vi "push_number.vi"(8 "error in (no error)":errorcluster, 10 "value":dbl, 11 "Lua in":refnum<class "Lua.lvclass">) -> (0 "error out":errorcluster, 3 "Lua out":refnum<class "Lua.lvclass">)   [LabVIEW 2020, in "Lua for LabVIEW.lvlib" / "Lua.lvclass"]
doc: "Push a numeric value to the Lua stack."
uses:
  Lua.lvclass
  Lua.lvclass/Lua.ctl
  lib/lua.dll/types/lua_error_code_offset.vi
  <vilib>/Utility/error.llb/Error Cluster From Error Code.vi
  lib/lua.dll/lua_pushnumber.vi
  lib/lua.dll/lua.dll.lvlib
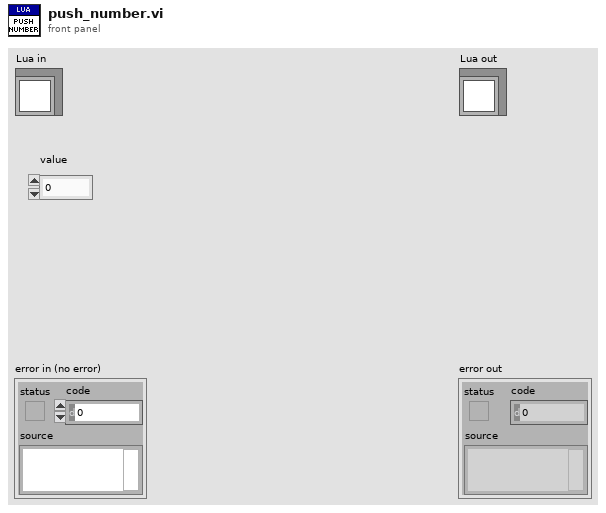
[diagram p1: front panel]
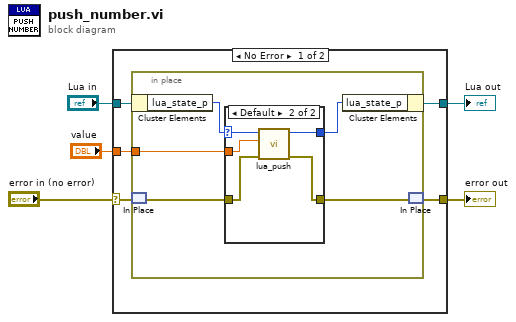
[diagram p0: block diagram]
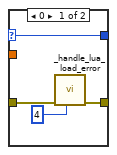
[diagram p2: hidden frame]
diagram:
  n1 = case shown="No Error" "error in (no error)" {
    selector: "error in (no error)" -> [w7 w26]
    tunnel: [w8 w26] -> w4
    tunnel: [w9 w25] -> w2
    tunnel: "Lua in" -> [w10 w25]
    tunnel: "value" -> [w6 _]
    frame No Error {
      n2 = in-place {
        in-place-border: w6 -> [w11]
        n3 = in-place-cluster #1(w10) -> ("lua_state_p"=w14:u64)
        n4 = in-place-match #2(w7) -> (w13:errorcluster)
        n5 = case shown="Default" w14 {
          selector: w14 -> [w19 w23]
          tunnel: [w19 w24] -> w15
          tunnel: w13 -> [w16 w22]
          tunnel: [w17 w21] -> w12
          tunnel: w11 -> [_ w20]
          frame 0 {
            n6 = call "_handle_lua_load_error.vi"("lua_load errcode"=4, "error in (no error)"=w16) -> ("error out"=w17:errorcluster)  [unwired: 9 in]
          }
          frame Default {
            n7 = call-poly "lua_push.vi"("error in (no error)"=w22, "Numeric"=w20, "lua_state_p"=w23) -> ("error out"=w21:errorcluster, "lua_state_p out"=w24:u64)  [unwired: 7 in]
          }
        }
        n8 = in-place-cluster #1("lua_state_p"=w15) -> (w9:refnum<class "Lua.lvclass">)
        n9 = in-place-match #2(w12) -> (w8:errorcluster)
      }
    }
    frame Error {
    }
  }
  "error out" <- w4
  "Lua out" <- w2
